vi "workspace.get_default.vi"(8 "error in":errorcluster, 11 "Nominal Client in":refnum<class "Nominal Client.lvclass">) -> (0 "error out":errorcluster, 1 "Workspace Details":T1, 2 "Workspace RID":string, 3 "Nominal Client out":refnum<class "Nominal Client.lvclass">)   [LabVIEW 2020, in "Nominal Client.lvclass"]
doc: "Gets the default workspace for the requesting user. If the user belongs to a single workspace,\nthat workspace is returned. Otherwise, if the user's organization has a default workspace and\nthe user belongs to it, that will be returned."
uses:
  Nominal Client.lvclass
  ce527530-f409-488f-b07f-3b5ecba8805e.vi
  <vilib>/JDP Science/JSONtext/JSON text to Variant.vi
  <vilib>/JDP Science/JSONtext/LVClass Serializer/JSONtext LVClass Serializer.lvclass
  Nominal Client.lvclass/Nominal Client.ctl
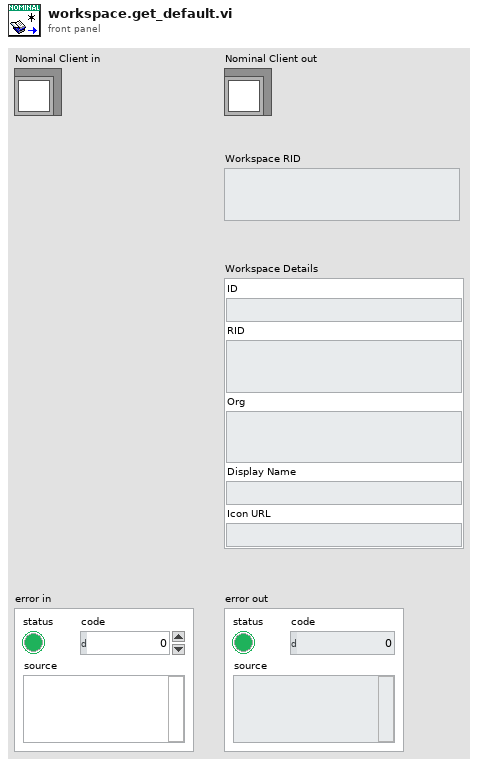
[diagram p1: front panel]
types:
  T1 = cluster{"ID":string, "RID":string, "Org":string, "Display Name":string, "Icon URL":string}
  T2 = cluster{"id":string, "rid":string, "org":string, "displayName":string, "iconUrl":string}
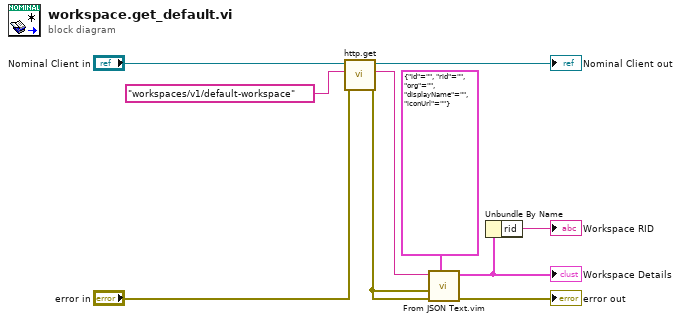
[diagram p0: block diagram]
diagram:
  n1 = call "http.get.vi"("error in"="error in", "Path"="workspaces/v1/default-workspace", "Nominal Client in"="Nominal Client in") -> ("error out"=w5:errorcluster, "Response"=w6:string, "Nominal Client out"=→"Nominal Client out":refnum<class "Nominal Client.lvclass">)  [unwired: 5 in, 1 out]
  "error out" <- w5
  n2 = call "From JSON Text.vim"("Data Type and Default Value"=T2 {"id"="", "rid"="", "org"="", "displayName"="", "iconUrl"=""} ("Workspace"), "error in (no error)"=w5, "JSON"=w6) -> ("Data out"=w2:T2)  [unwired: 7 in, 1 out]
  "Workspace Details" <- w2
  n3 = Unbundle By Name(w2) -> ("rid"=→"Workspace RID":string)
